vi "Axis Manager.vi"() -> ()   [LabVIEW 2014]
uses:
  Axis config.ctl
  Axis enum.ctl
panel:
  out "Detected stages":i32(listbox)
  out "Multicolumn Listbox":i32(listbox)
  out "Config":T1[](array[typedef])
  in  "Stage":u16(ring) items=["C", "E"]
  # "Configuration"
  # "LabVIEW Example"
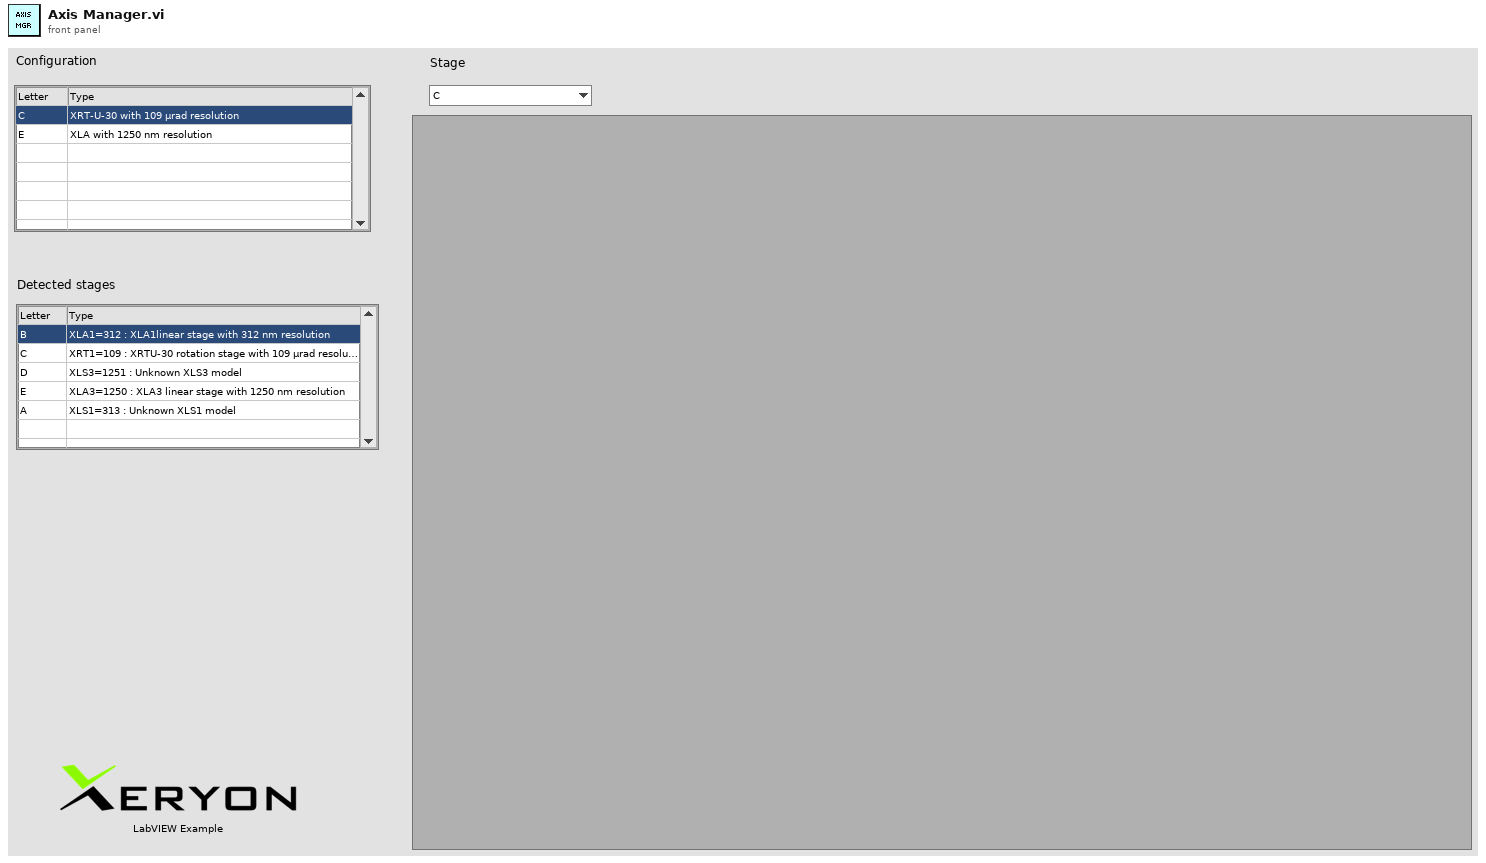
[diagram p1: front panel]
types:
  T1 = typedef "Axis config.ctl" = cluster{"Letter":string, "Stagetype":T2}
  T2 = typedef "Axis enum.ctl" = enum16{"XLA with 50 µm resolution", "XLA with 10 µm resolution", "XLA with 1250 nm resolution", "XLA with 312 nm resolution", "XLA with 78 nm resolution", "XLS with 1250 nm resolution", "XLS with 312 nm resolution", "XLS with 78nm resolution", "XLS with 5nm resolution", "XLS with 1 nm resolution", "XRT-A with 109 µrad resolution", "XRT-U-30 with 109 µrad resolution", "XRT-U-30 with 49 µrad resolution", "XRT-U-30 with 19 µrad resolution", "XRT-U-30 with 3 µrad resolution", "XRT-U-40 with 109 µrad resolution", "XRT-U 40 with 49 µrad resolution", "XRT-U-40 with 19 µrad resolution", "XRT-U-40 with 3 µrad resolution", "XRT-U-60 with 109 µrad resolution", "XRT-U-60 with 49 µrad resolution", "XRT-U-60 with 19 µrad resolution", "XRT-U-60 with 3 µrad resolution"}
  T3 = enum16{"Init", "Set stage data", "Update position", "Get"}
  T4 = cluster{"Drive letter":string, "Drive type":T2}[]
  T5 = typedef "Serial parameters.ctl" = enum16{"Serial number", "Software number", "Type of stage", "Status", "Frequency", "Encoder position", "Desired position", "Info", "Phase correction", "Timestamp", "Proportional control factor", "Sync", "XRT1", "XRT3", "XRTA", "XLS1", "XLS3", "XLA1", "XLA3"}
  T6 = cluster{"Parameters out":T5[], "Values out":i32[], "Stage type":string, "Stage letter":string}[]
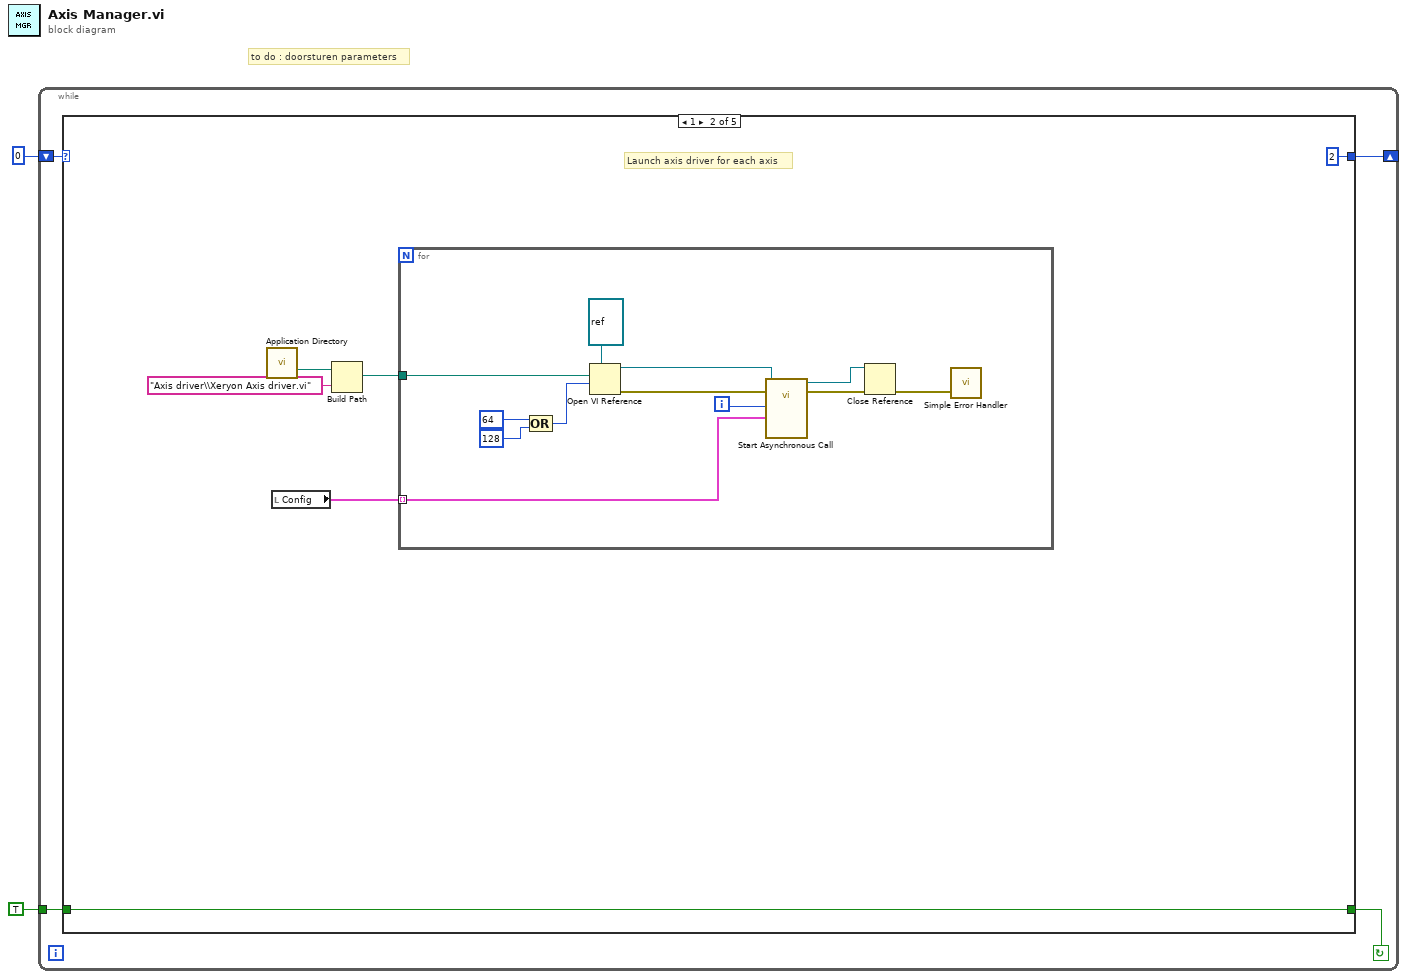
[diagram p0: block diagram]
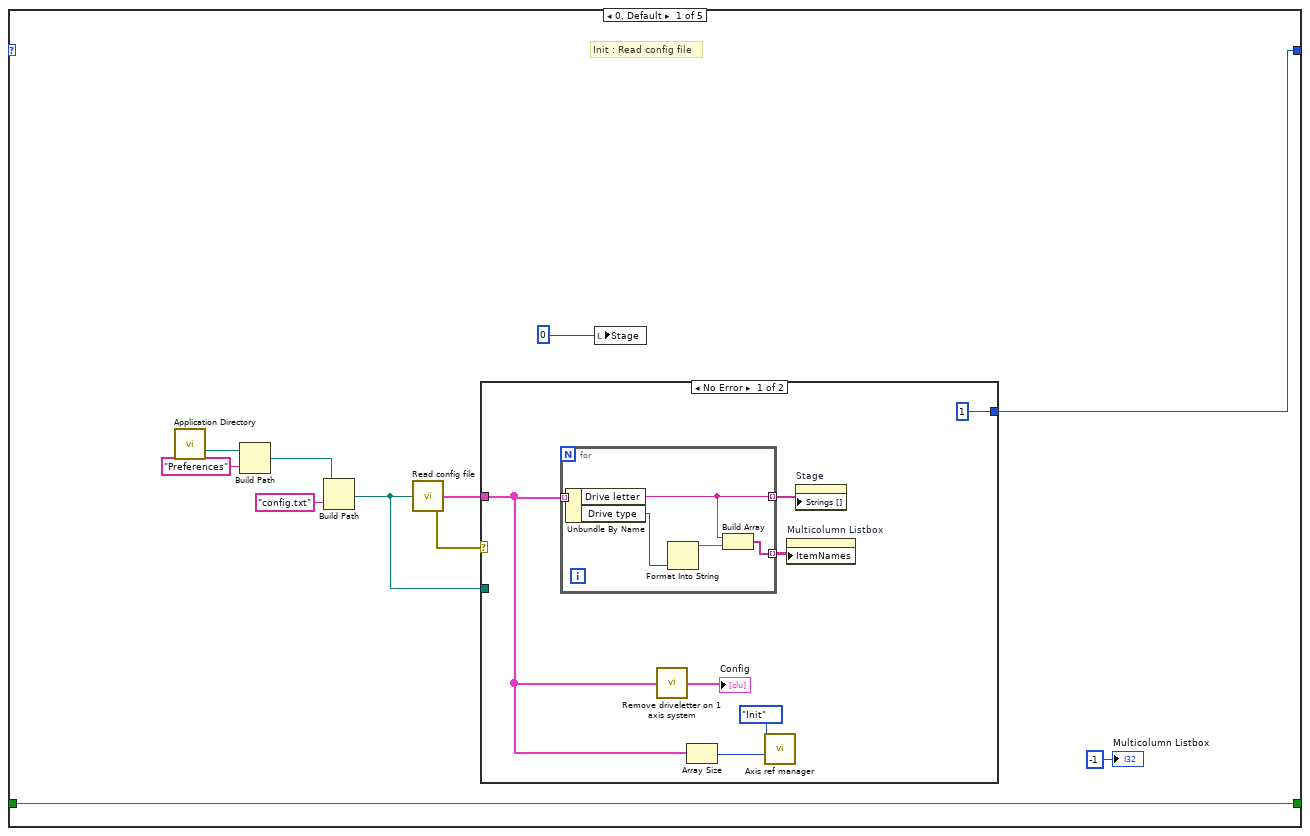
[diagram p2: hidden frame]
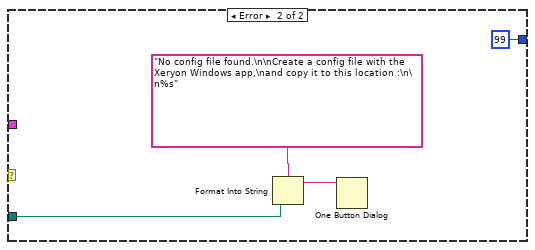
[diagram p3: hidden frame]
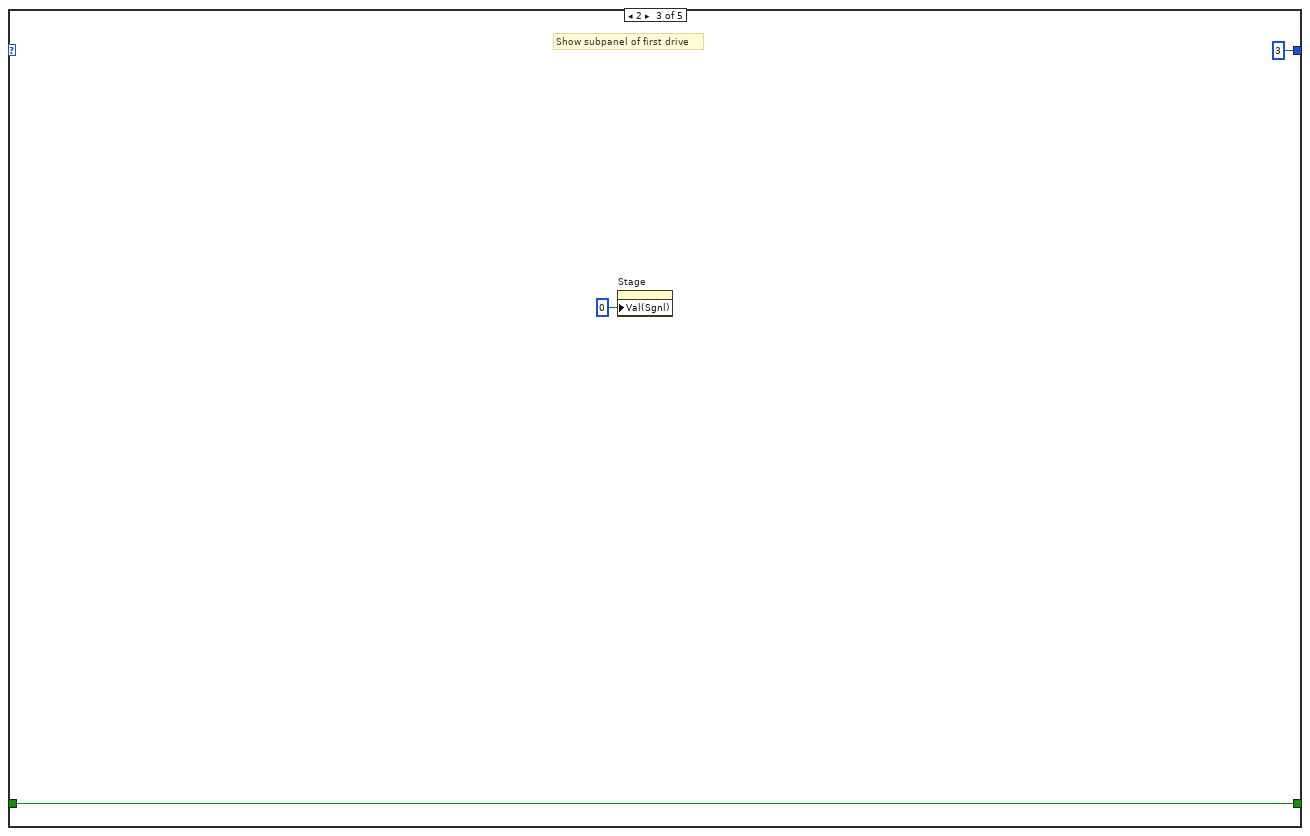
[diagram p4: hidden frame]
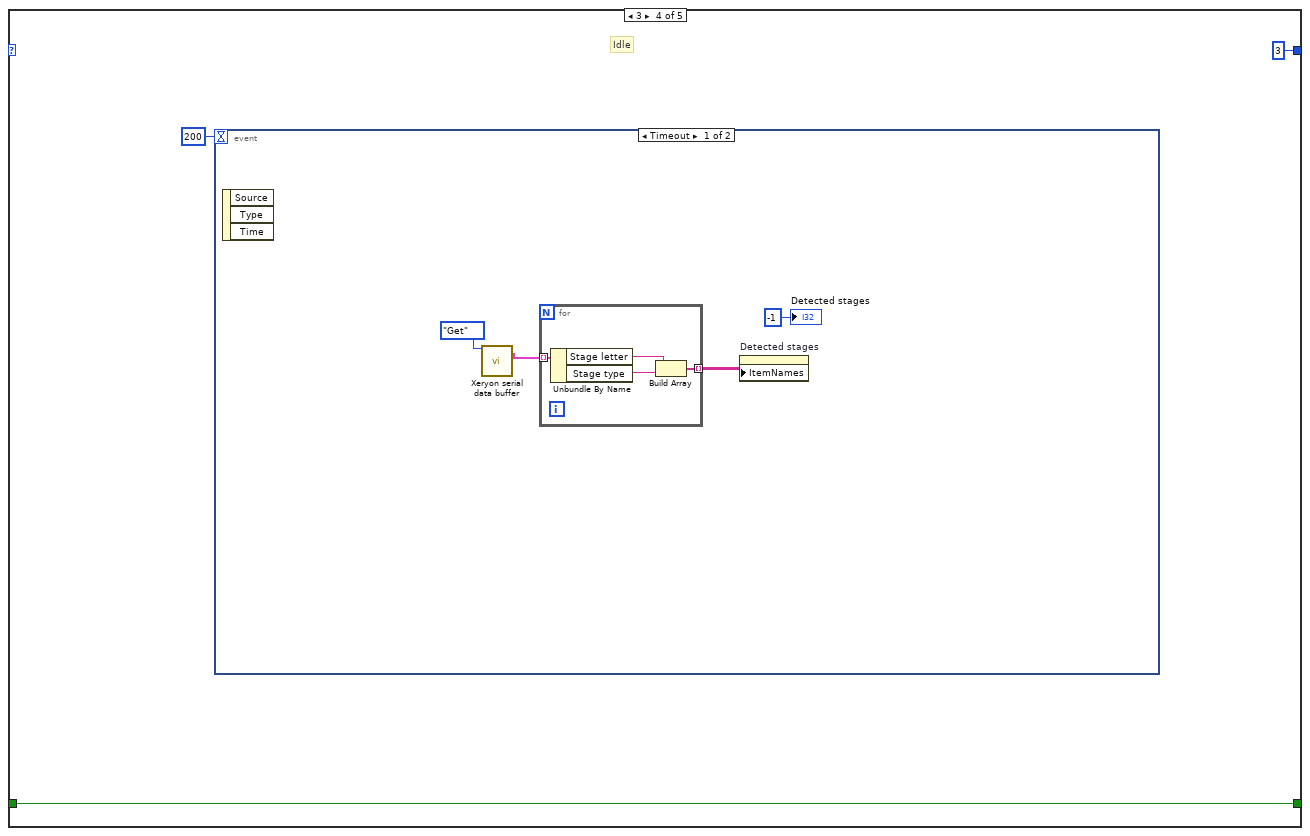
[diagram p5: hidden frame]
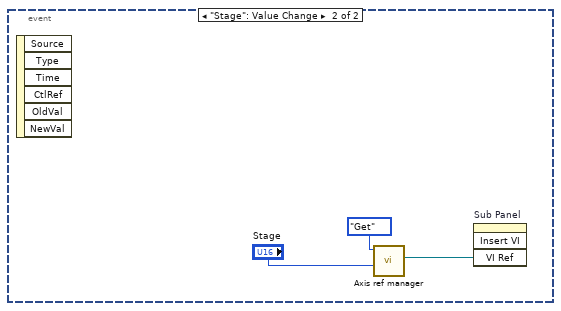
[diagram p6: hidden frame]
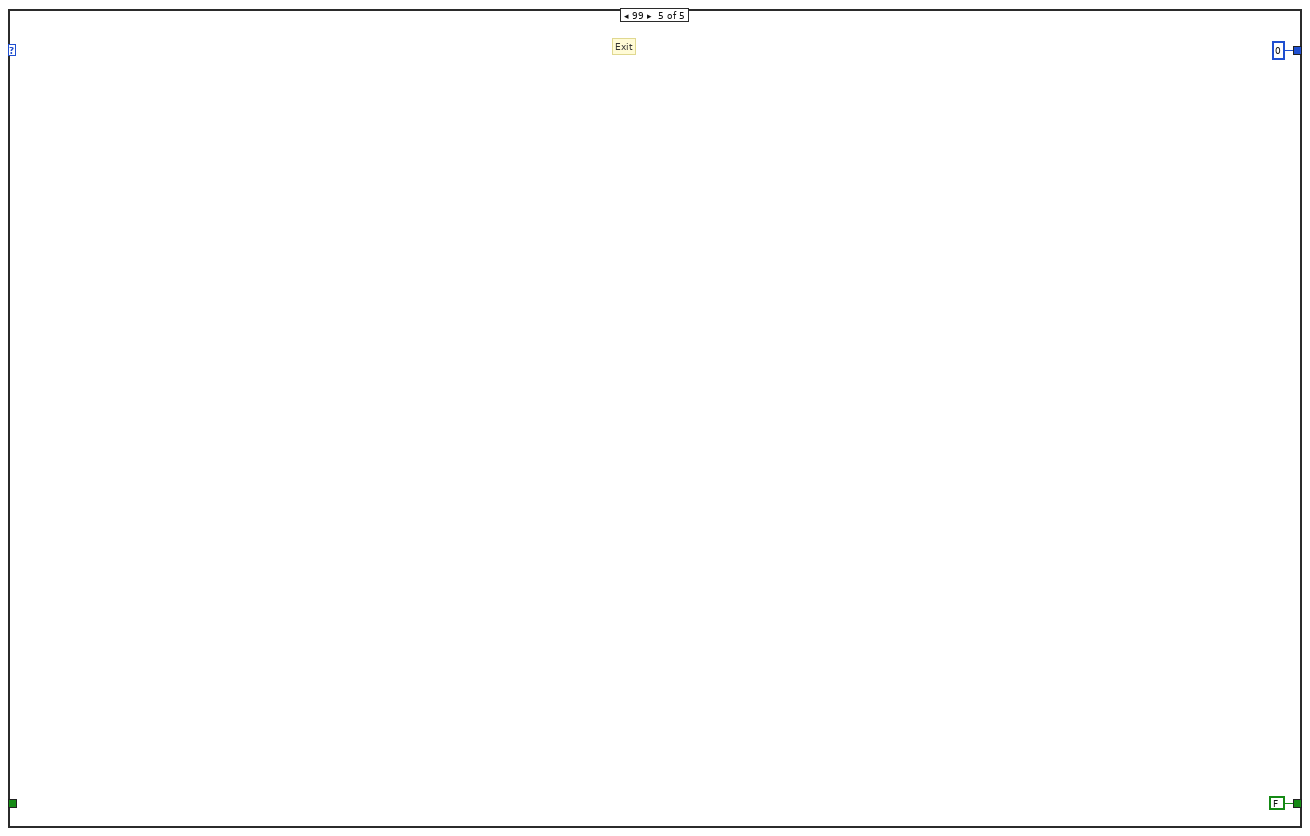
[diagram p7: hidden frame]
diagram:
  # "to do : doorsturen parameters"
  n1 = while {
    shift-right: [w3] -> _
    shift-left: 0 -> [w6]
    tunnel: TRUE -> [w5]
    stop <- w4 continue-if-true
    n2 = case shown="1" w6 {
      tunnel: [w13 w38 w53 w57 FALSE] -> w4
      tunnel: w5 -> [w13 w38 w53 w57 _]
      tunnel: [w9 2 3 3 0] -> w3
      frame 0, Default {
        # "Init : Read config file"
        n3 = call <vilib>:"Application Directory.vi"() -> ("Application Directory"=w17:path)
        n4 = Build Path(base path=w17, name or relative path="Preferences") -> (appended path=w15:path)
        n5 = Build Path(base path=w15, name or relative path="config.txt") -> (appended path=w10:path)
        n6 = call "Read config file.vi"("file (use dialog)"=w10) -> ("error out"=w11:errorcluster, "Drives"=w7:T4)  [unwired: 3 in]
        n7 = case shown="No Error" w11 {
          tunnel: w7 -> [w18 _]
          tunnel: w10 -> [_ w31]
          tunnel: [1 99] -> w9
          frame No Error {
            n8 = for {
              tunnel: w18 -> [w29] mode=indexing
              tunnel: [w27] -> w24 mode=indexing
              tunnel: [w28] -> w20 mode=indexing
              n9 = Unbundle By Name(w29) -> ("Drive letter"=w27:string, "Drive type"=w26:T2)
              n10 = Format Into String(w26) -> (resulting string=w25:string)  [unwired: 3 in, 1 out]
              n11 = Build Array(w27, w25) -> (w28:string[])
            }
            n12 = call "Remove driveletter on 1 axis system.vi"("Config in"=w18) -> ("Config out"=→"Config":T4)  [unwired: 4 in]
            n13 = Array Size(array=w18) -> (size(s)=w21:i32)
            n14 = call "Axis ref manager.vi"("Index/size in"=w21, "Mode"=enum16{"Init", "Set", "Get"}."Init") -> ()  [unwired: 5 in, 1 out]
            n15 = property on="Multicolumn Listbox" class="MCListbox (strict)"("ItemNames"=w20) -> ()  [unwired: 2 in, 2 out]
            n16 = property on="Stage" class="Ring (strict)"("Strings []"=w24) -> ()  [unwired: 2 in, 2 out]
          }
          frame Error {
            n17 = Format Into String(format string="No config file found.\n\nCreate a config file with the Xeryon Windows app,\nand copy it to this location :\n\n%s" ("message"), w31) -> (resulting string=w32:string)  [unwired: 2 in, 1 out]
            n18 = One Button Dialog(message=w32) -> ()  [unwired: 1 in, 1 out]
          }
        }
        n19 = local write "Stage"(0) -> ()
        "Multicolumn Listbox" <- -1 ("Multicolumn Listbox")
      }
      frame 1 {
        # "Launch axis driver for each axis"
        n20 = call <vilib>:"Application Directory.vi"() -> ("Application Directory"=w36:path)
        n21 = local read "Config"() -> (w37:T1[])
        n22 = Build Path(base path=w36, name or relative path="Axis driver\\Xeryon Axis driver.vi") -> (appended path=w34:path)
        n23 = for {
          tunnel: w37 -> [w40] mode=indexing
          tunnel: w34 -> [w41]
          i -> [w43]
          n24 = Compound Arithmetic op=OR(64, 128) -> (w51:i32)
          n25 = Open VI Reference(type specifier VI Refnum (for type only)=refnum<vi> refnum, vi path=w41, options=w51) -> (vi reference=w44:refnum<vi>, error out=w50:errorcluster)  [unwired: 3 in]
          n26 = call-by-ref "Start Asynchronous Call"(reference=w44, error in=w50, "Config"=w40, "Stage index"=w43) -> (reference out=w47:refnum<vi>, error out=w46:errorcluster)  [unwired: 4 in]
          n27 = Close Reference(reference=w47, error in (no error)=w46) -> (error out=w42:errorcluster)
          n28 = call <vilib>:"Simple Error Handler.vi"("error in (no error)"=w42) -> ()  [unwired: 4 in, 5 out]
        }
      }
      frame 2 {
        # "Show subpanel of first drive"
        n29 = property on="Stage" class="Ring (strict)"("Val(Sgnl)"=u16 0 ("Value (Signaling)")) -> ()  [unwired: 2 in, 2 out]
      }
      frame 3 {
        # "Idle"
        n30 = event shown="[0] Timeout" {
          selector: _ -> [_ _]
          dyn-events: _ -> [_ _]
          timeout: 200 -> [_ _]
          event Timeout {
            n31 = event-data() -> ()  [unwired: 1 in, 3 out]
            n32 = call "Xeryon serial data buffer.vi"("Mode"=T3."Get") -> ("Stage data"=w58:T6)  [unwired: 8 in, 6 out]
            n33 = for {
              tunnel: w58 -> [w65] mode=indexing
              tunnel: [w62] -> w61 mode=indexing
              n34 = Unbundle By Name(w65) -> ("Stage letter"=w64:string, "Stage type"=w63:string)
              n35 = Build Array(w64, w63) -> (w62:string[])
            }
            n36 = property on="Detected stages" class="MCListbox (strict)"("ItemNames"=w61) -> ()  [unwired: 2 in, 2 out]
            "Detected stages" <- -1 ("Detected stages")
          }
          event "Stage": Value Change {
            n37 = event-data() -> ()  [unwired: 1 in, 6 out]
            n38 = call "Axis ref manager.vi"("Index/size in"="Stage", "Mode"=enum16{"Init", "Set", "Get"}."Get") -> ("Ref out"=w67:refnum<vi>)  [unwired: 5 in]
            n39 = invoke on="Sub Panel" class="SubPnl" method="Insert VI"("VI Ref"=w67) -> ()  [unwired: 3 in, 4 out]
          }
        }
      }
      frame 99 {
        # "Exit"
      }
    }
  }
